vi "Read-exec-script.vi"(8 "error in":errorcluster, 11 "file (use dialog)":path) -> (0 "error out":errorcluster, 2 "Commands Str Array":string[][](array[string]), 3 "Commands":T1[](array[typedef]))   [LabVIEW 2021]
uses:
  Controls/Command_Enum.ctl
  Controls/Command_cluster.ctl
panel:
  in  "Commands":T2=enum."Y Home"
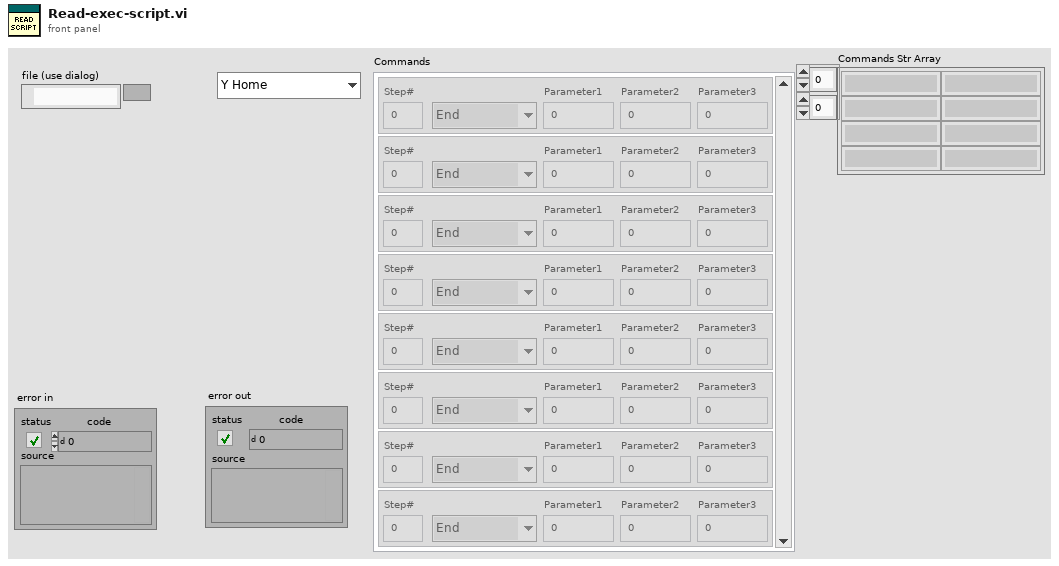
[diagram p1: front panel]
types:
  T1 = typedef "Command_cluster.ctl" = cluster{"Step#":dbl, "Commands":T2, "Parameter1":dbl, "Parameter2":dbl, "Parameter3":dbl}
  T2 = typedef "Command_Enum.ctl" = enum16{"End", "Home All", "X Home", "Y Home", "X Move Rel", "X Move Abs", "Y Move Rel", "Y Move Abs", "Wait", "Repeat", "Reset Intlk Timer", "Laser Sys ON", "Laser ENA"}
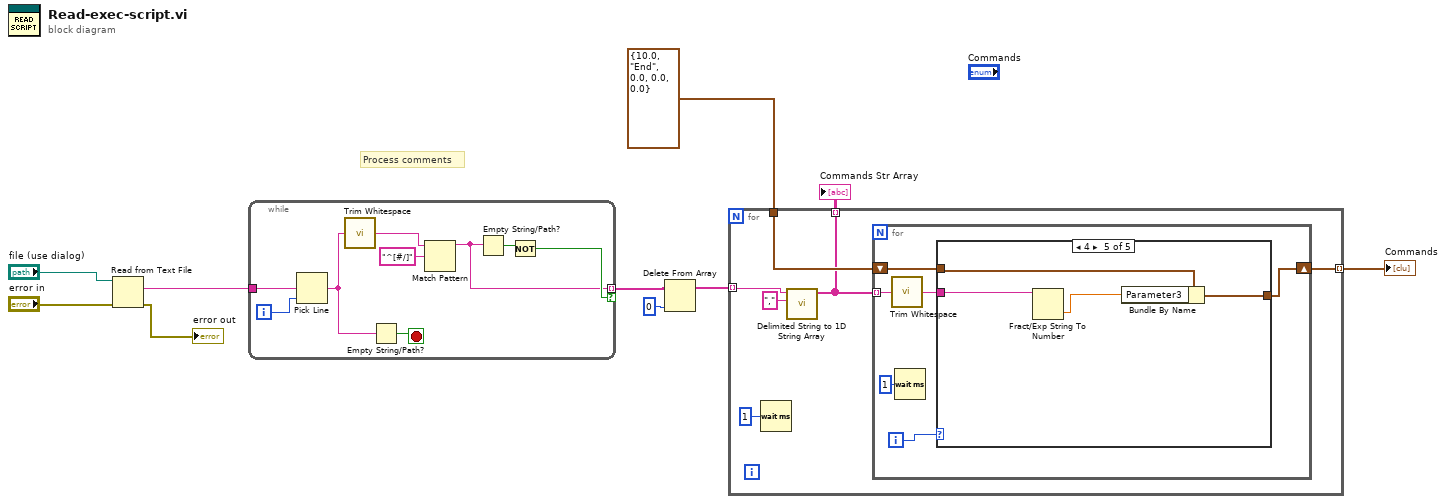
[diagram p0: block diagram]
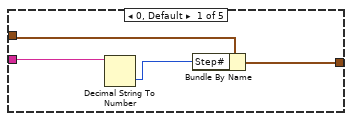
[diagram p2: hidden frame]
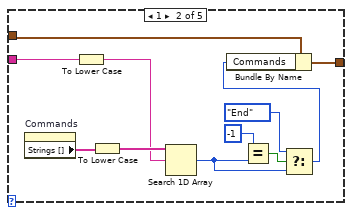
[diagram p3: hidden frame]
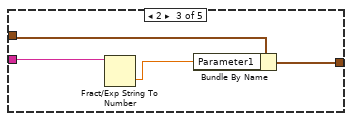
[diagram p4: hidden frame]
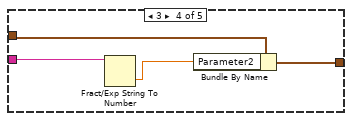
[diagram p5: hidden frame]
diagram:
  # "Process comments"
  n1 = Read from Text File(file (use dialog)="file (use dialog)", error in="error in") -> (text=w10:string, error out=→"error out":errorcluster)  [unwired: 2 in, 2 out]
  n2 = while {
    tunnel: w10 -> [w19]
    tunnel: [w11] -> w2 mode=indexing if=w14
    i -> [w18]
    stop <- w17 stop-if-true
    n3 = Pick Line(multi-line string=w19, line index=w18) -> (output string=w13:string)  [unwired: 1 in]
    n4 = call <vilib>:"Trim Whitespace.vi"("string"=w13) -> ("trimmed string"=w12:string)  [unwired: 1 in]
    n5 = Empty String/Path?(string/path=w13) -> (empty?=w17:bool)
    n6 = Match Pattern(string=w12, regular expression="^[#/]") -> (before substring=w11:string)  [unwired: 1 in, 3 out]
    n7 = Empty String/Path?(string/path=w11) -> (empty?=w15:bool)
    n8 = Not(x=w15) -> (.not. x?=w14:bool)
  }
  n9 = Delete From Array(array=w2, index=0) -> (array with subset deleted=w8:string[])  [unwired: 1 in, 1 out]
  n10 = for {
    tunnel: w8 -> [w24] mode=indexing
    tunnel: T1 {"Step#"=10.0, "Commands"=enum."End", "Parameter1"=0.0, "Parameter2"=0.0, "Parameter3"=0.0} ("Cmd element") -> [w23]
    tunnel: [w22] -> w6 mode=indexing
    tunnel: [w20] -> w1 mode=indexing
    n11 = Wait (ms)(milliseconds to wait=u32 1) -> ()  [unwired: 1 out]
    n12 = call <vilib>:"Delimited String to 1D String Array.vi"("delimiter"=",", "delimited string"=w24) -> ("string array"=w20:string[])  [unwired: 9 in]
    n13 = for {
      tunnel: w20 -> [w28] mode=indexing
      shift-right: [w29] -> w22
      shift-left: w23 -> [w31]
      i -> [w30]
      n14 = call <vilib>:"Trim Whitespace.vi"("string"=w28) -> ("trimmed string"=w27:string)  [unwired: 1 in]
      n15 = Wait (ms)(milliseconds to wait=u32 1) -> ()  [unwired: 1 out]
      n16 = case shown="4" w30 {
        tunnel: w31 -> [w35 w46 w50 w54 w58]
        tunnel: w27 -> [w34 w37 w49 w53 w57]
        tunnel: [w32 w45 w47 w51 w55] -> w29
        frame 0, Default {
          n17 = Decimal String To Number(string=w34) -> (number=w33:i32)  [unwired: 2 in, 1 out]
          n18 = Bundle By Name(cluster=w35, "Step#"=w33) -> (w32:T1)
        }
        frame 1 {
          n19 = property on="Commands" class="Enum (strict)"() -> ("Strings []"=w39:string[])  [unwired: 2 in, 2 out]
          n20 = To Lower Case(string=w37) -> (all lower case string=w36:string)
          n21 = To Lower Case(string=w39) -> (all lower case string=w38:string[])
          n22 = Search 1D Array(1D array=w38, element=w36) -> (index of element=w42:i32)  [unwired: 1 in]
          n23 = Equal?(x=-1 ("y"), y=w42) -> (x = y?=w44:bool)
          n24 = Select(t=Command_Enum."End" ("Commands"), s=w44, f=w42) -> (s? t:f=w40:i32)
          n25 = Bundle By Name(cluster=w46, "Commands"=w40) -> (w45:T1)
        }
        frame 2 {
          n26 = Fract/Exp String To Number(string=w49) -> (number=w48:dbl)  [unwired: 3 in, 1 out]
          n27 = Bundle By Name(cluster=w50, "Parameter1"=w48) -> (w47:T1)
        }
        frame 3 {
          n28 = Fract/Exp String To Number(string=w53) -> (number=w52:dbl)  [unwired: 3 in, 1 out]
          n29 = Bundle By Name(cluster=w54, "Parameter2"=w52) -> (w51:T1)
        }
        frame 4 {
          n30 = Fract/Exp String To Number(string=w57) -> (number=w56:dbl)  [unwired: 3 in, 1 out]
          n31 = Bundle By Name(cluster=w58, "Parameter3"=w56) -> (w55:T1)
        }
      }
    }
  }
  "Commands" <- w6
  "Commands Str Array" <- w1
